vi "CleanVision.vi"(1 "Targets":dbl, 2 "Input":dbl[](array[numeric])) -> (0 "Output":dbl[][](array[numeric]))   [LabVIEW 2016]
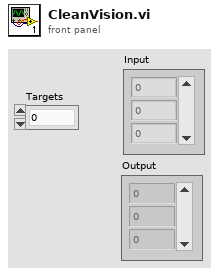
[diagram p1: front panel]
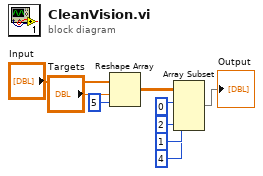
[diagram p0: block diagram]
diagram:
  n1 = Reshape Array("Input", "Targets", 5 ("dimension size")) -> (w6:dbl[][])
  n2 = Array Subset(array=w6, index (row)=0 ("index"), length (row)=2 ("length"), index (col)=1 ("index"), length (col)=4 ("length")) -> (→"Output":dbl[][])
